vi "ShowLifetimeAndF2Image.vi"(2 "Path":refnum<vi>, 5 "threshold (min)":u16, 6 "notes 2":refnum<vi>) -> ()   [LabVIEW 2009]
panel:
  in  "save tau":bool
  in  "channel":u16(ring) items=["sum", "1", "2", "3", "4", "5", "6", "7", "8"]
  in  "draw F2 image":bool caption="display F2 image"
  in  "display tau image":bool
  in  "Color Palette F2-image":T1(ring)
  in  "min. F2 Value":sgl min=0 max=1 format="%.2f"
  in  "max. F2 Value":sgl=1.0 min=0 max=1 format="%.2f"
  in  "min. tau Value":dbl min=0.0 format="%.2f"
  in  "max. tau Value":dbl=10.0 min=0.0 format="%.2f"
  in  "Color Palette lifetime":T1(ring)
  in  "notes":string
  out "Ampel":cluster{"RED":bool, "YELLOW":bool, "GREEN":bool}
  in  "F2-channel":u8=2 min=1 max=16 step=1
  in  "Export":bool
  in  "stop":bool
  in  "plane":i32
  # "t"
  # "Fx"
  # "channel"
  # "S channel"
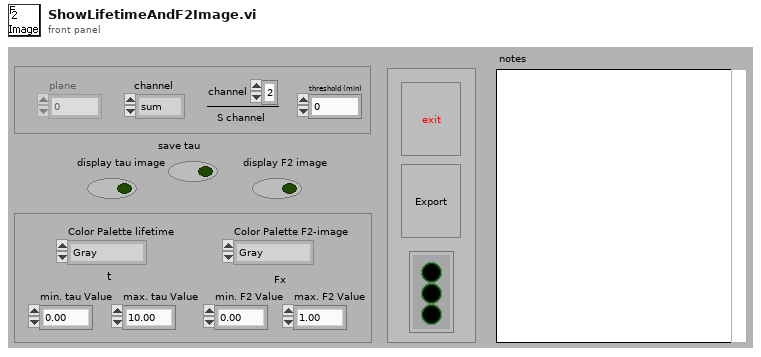
[diagram p1: front panel]
types:
  T1 = enum32{"Gray", "Binary", "Gradient", "Rainbow", "Temperature"}
  T2 = enum16{"create", "Input", "draw", "colorpal", "dump", "Get"}
  T3 = enum16{"create", "Input", "draw", "colorpal", "dump"}
  T4 = enum16{"ini", "get", "change", "export", "draw", "dump", "kill", "colorpal"}
  T5 = enum16{"create", "Input", "draw", "colorpal", "dump", "Get", "kill"}
  T6 = enum16{"create", "Input", "draw", "colorpal", "dump", "get", "kill"}
  T7 = enum16{"create", "Input", "draw", "colorpal", "dump", "get"}
  T8 = typedef "Settings.ctl" = cluster{"threshold":cluster{"max":u32, "min":u32}, "RGB or false color":bool, "16bit":bool, "log/lin axis":u16, "spotsize button":bool, "Pixelsize":u16, "autoscale x":bool, "autoscale y":bool, "correlation":bool, "ADC-Resolution":i32, "F2-lifetime":cluster{"display tau":bool, "display F2":bool, "Palette Number lifetime":enum32{"Gray", "Binary", "Gradient", "Rainbow", "Temperature"}, "Palette Number F2":enum32{"Gray", "Binary", "Gradient", "Rainbow", "Temperature"}, "max tau-Value":dbl, "min tau-Value":dbl, "max F2-Value":dbl, "min F2-Value":dbl}, "TAC-Window 1":u16, "TAC-Window 2":u16, "false color palette":cluster{"1":u32, "2":u32, "3":u32, "4":u32, "5":u32, "6":u32, "7":u32, "8":u32, "8 2":u32, "8 3":u32, "8 4":u32, "8 5":u32}}
  T9 = typedef "FIFOSettings_BH.ctt" = cluster{"Measurement":cluster{"Binning (ms)":sgl, "External Trigger Condition":u16, "Stop Condition:":u16, "Stop Count":dbl, "Buffer Size (Photons)":u16, "No of Channels":u16, "Ext Latch Delay":i16}, "ADC":cluster{"Module":u16, "ADC Resolution":i32, "Dither Range":i16, "Count Increment":i16, "Macro Time Clock":i16}, "SYNC":cluster{"SYNC ZC Level (mV)":sgl, "SYNC Freq Divider":i16, "SYNC Holdoff (ns)":sgl, "SYNC Threshold (mV)":sgl}, "TAC":cluster{"TAC Range (ns)":sgl, "TAC Gain":i16, "TAC Offset (%)":sgl, "TAC Limit Low (%)":sgl, "TAC Limit High (%)":sgl}, "CFD":cluster{"CFD Limit Low (mV)":sgl, "CFD Limit High (mV)":sgl, "CFD ZC Level (mV)":sgl, "CFD Holdoff (ns)":sgl}}
  T10 = typedef "ImageSettings.ctt" = cluster{"Start Position (µm)":cluster{"x":dbl, "y":dbl, "z":dbl}, "End Position (µm)":cluster{"x":dbl, "y":dbl, "z":dbl}, "Image Resolution (nm/pixel)":cluster{"x":dbl, "y":dbl, "z":dbl}, "Image Size (µm)":cluster{"x":dbl, "y":dbl, "z":dbl}, "Image Size (pixel)":cluster{"x":u32, "y":u32, "z":u32}, "Time Resolution\n(ms/pixel)":dbl, "1st Axis":u16, "2nd Axis":u16, "Retrace":bool, "Estimated Time":string}
  T11 = typedef "IMAQ Image.ctl" = refnum<image>
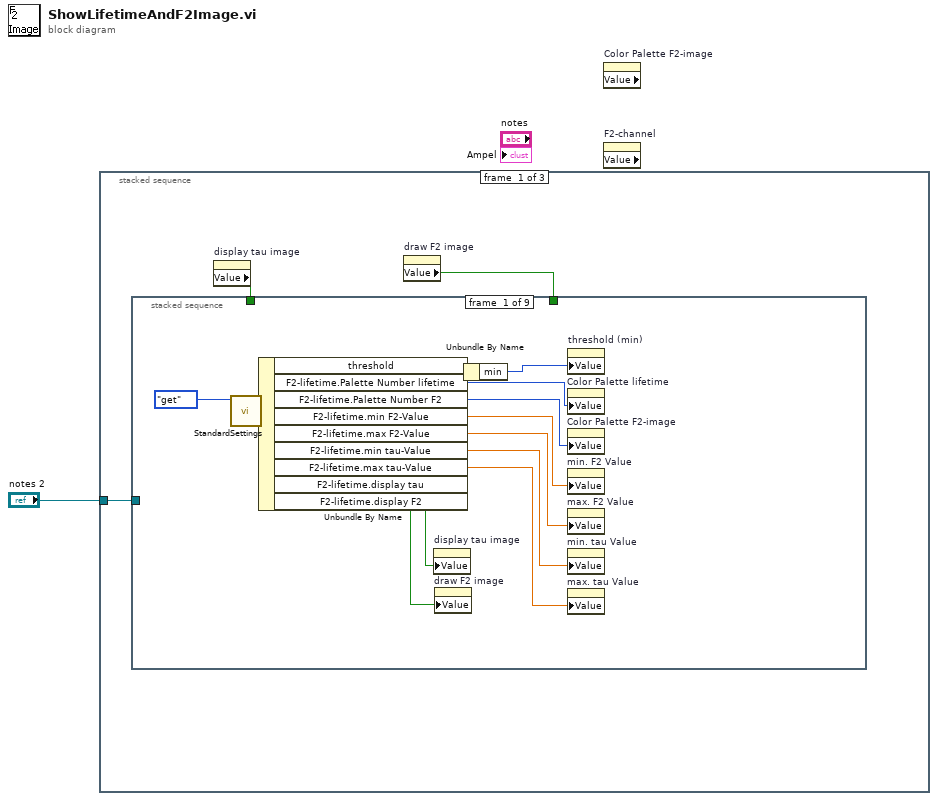
[diagram p0: block diagram]
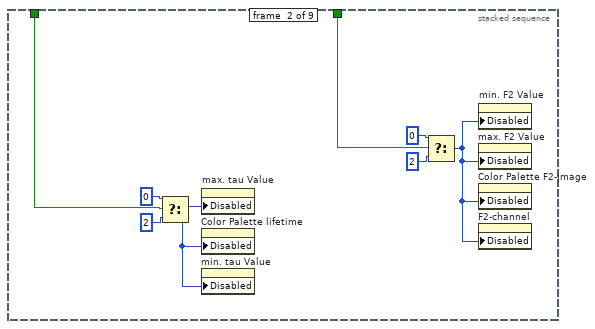
[diagram p2: hidden frame]
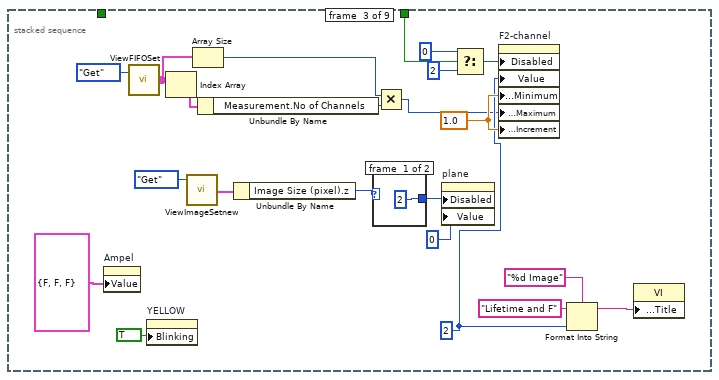
[diagram p3: hidden frame]
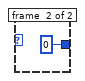
[diagram p4: hidden frame]
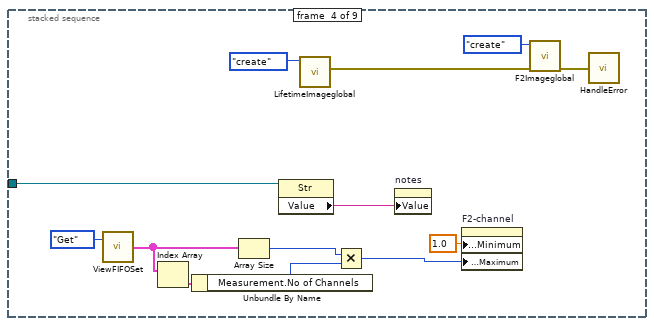
[diagram p5: hidden frame]
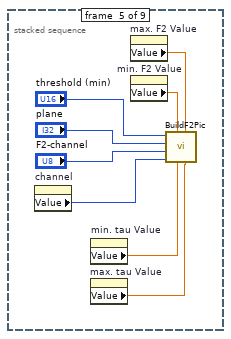
[diagram p6: hidden frame]
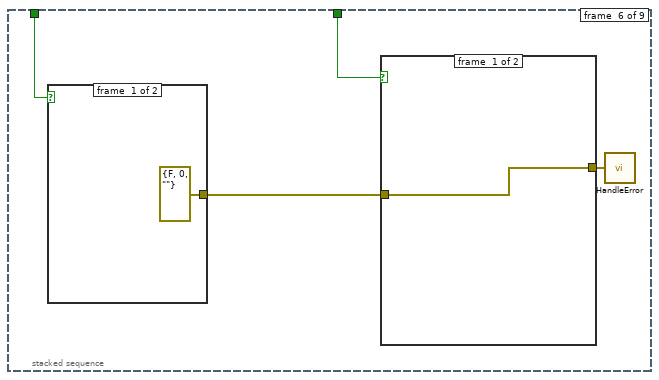
[diagram p7: hidden frame]
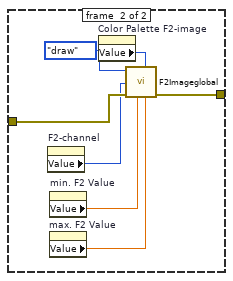
[diagram p8: hidden frame]
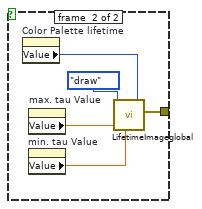
[diagram p9: hidden frame]
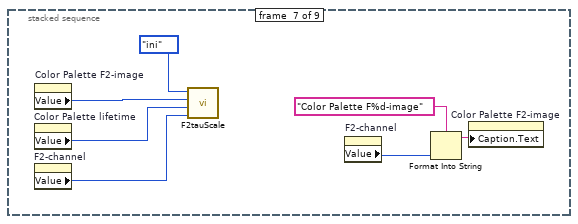
[diagram p10: hidden frame]
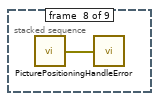
[diagram p11: hidden frame]
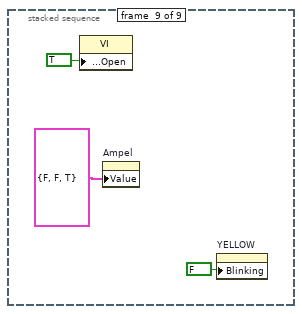
[diagram p12: hidden frame]
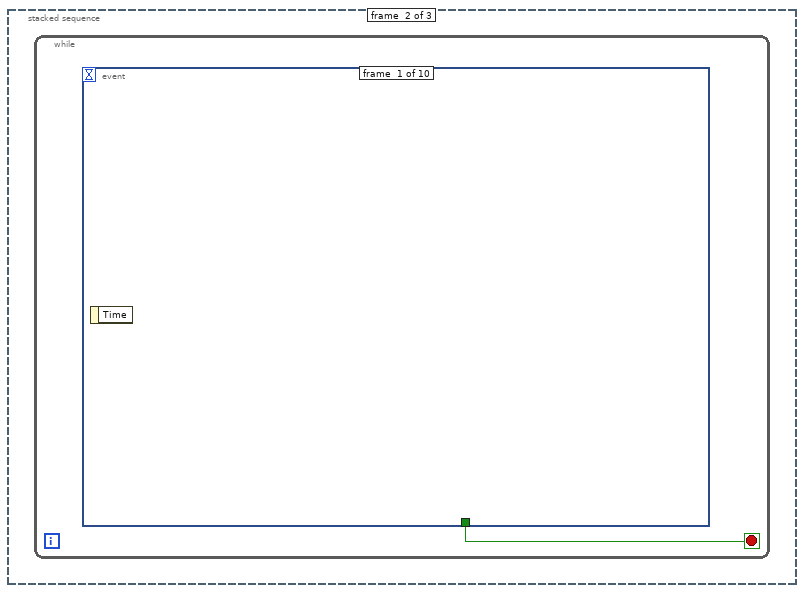
[diagram p13: hidden frame]
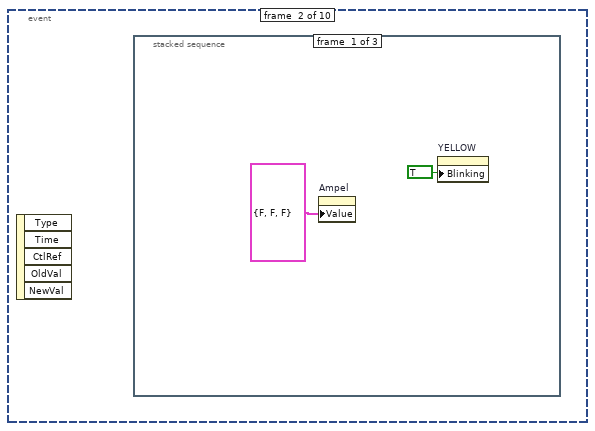
[diagram p14: hidden frame]
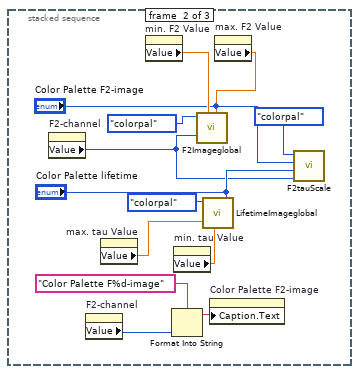
[diagram p15: hidden frame]
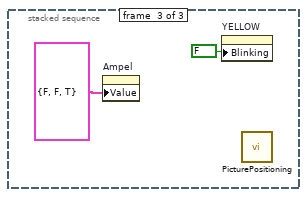
[diagram p16: hidden frame]
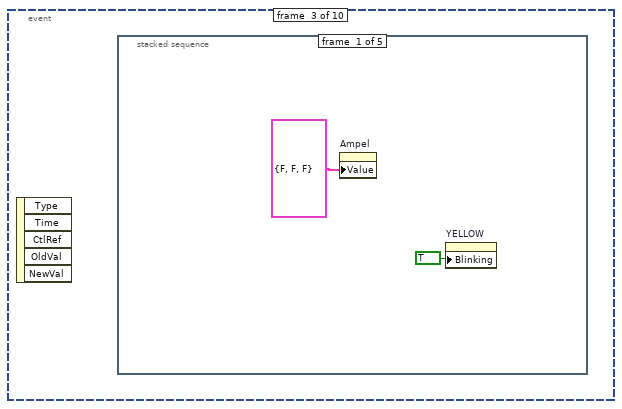
[diagram p17: hidden frame]
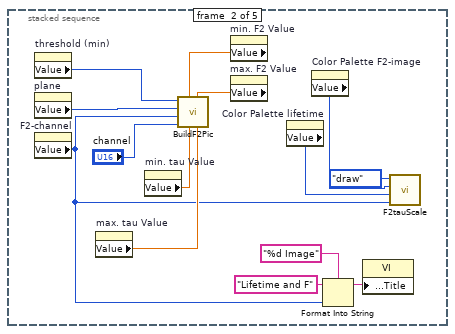
[diagram p18: hidden frame]
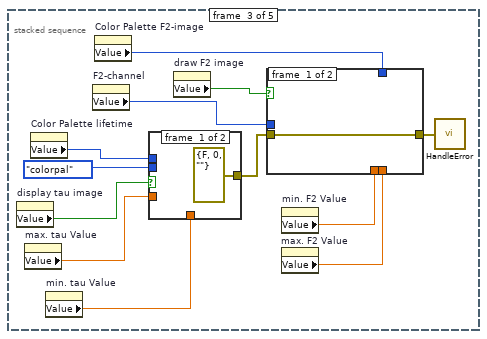
[diagram p19: hidden frame]
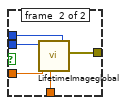
[diagram p20: hidden frame]
diagram:
  n1 = stacked-sequence {
    tunnel: "notes 2" -> [w4 _ w350]
    frame #0 {
      n2 = property on="display tau image" class="Bool (strict)"() -> ("Value"=w3:bool)  [unwired: 2 in, 2 out]
      n3 = property on="draw F2 image" class="Bool (strict)"() -> ("Value"=w2:bool)  [unwired: 2 in, 2 out]
      n4 = stacked-sequence {
        tunnel: w4 -> [_ _ _ w56 _ _ _ _ _]
        tunnel: w3 -> [_ w18 _ _ _ w72 _ _ _]
        tunnel: w2 -> [_ w17 w31 _ _ w70 _ _ _]
        frame #0 {
          n5 = call "StandardSettings.vi"("Enum"=enum16{"Load", "get", "Save", "set"}."get") -> ("StandardSettings"=w15:T8)  [unwired: 4 in]
          n6 = Unbundle By Name(w15) -> ("threshold"=w6:cluster{"max":u32, "min":u32}, "F2-lifetime.Palette Number lifetime"=w14:T1, "F2-lifetime.Palette Number F2"=w13:T1, "F2-lifetime.min F2-Value"=w12:dbl, "F2-lifetime.max F2-Value"=w11:dbl, "F2-lifetime.min tau-Value"=w10:dbl, "F2-lifetime.max tau-Value"=w9:dbl, "F2-lifetime.display tau"=w8:bool, "F2-lifetime.display F2"=w7:bool)
          n7 = property on="display tau image" class="Bool (strict)"("Value"=w8) -> ()  [unwired: 2 in, 2 out]
          n8 = property on="draw F2 image" class="Bool (strict)"("Value"=w7) -> ()  [unwired: 2 in, 2 out]
          n9 = Unbundle By Name(w6) -> ("min"=w5:u32)
          n10 = property on="threshold (min)" class="DigNum (strict)"("Value"=w5) -> ()  [unwired: 2 in, 2 out]
          n11 = property on="Color Palette lifetime" class="Enum (strict)"("Value"=w14) -> ()  [unwired: 2 in, 2 out]
          n12 = property on="Color Palette F2-image" class="Enum (strict)"("Value"=w13) -> ()  [unwired: 2 in, 2 out]
          n13 = property on="min. F2 Value" class="DigNum (strict)"("Value"=w12) -> ()  [unwired: 2 in, 2 out]
          n14 = property on="max. F2 Value" class="DigNum (strict)"("Value"=w11) -> ()  [unwired: 2 in, 2 out]
          n15 = property on="min. tau Value" class="DigNum (strict)"("Value"=w10) -> ()  [unwired: 2 in, 2 out]
          n16 = property on="max. tau Value" class="DigNum (strict)"("Value"=w9) -> ()  [unwired: 2 in, 2 out]
        }
        frame #1 {
          n17 = Select(t=0, s=w18, f=2) -> (s? t:f=w19:i32)
          n18 = property on="max. tau Value" class="DigNum (strict)"("Disabled"=w19) -> ()  [unwired: 2 in, 2 out]
          n19 = property on="Color Palette lifetime" class="Enum (strict)"("Disabled"=w19) -> ()  [unwired: 2 in, 2 out]
          n20 = property on="min. tau Value" class="DigNum (strict)"("Disabled"=w19) -> ()  [unwired: 2 in, 2 out]
          n21 = Select(t=0, s=w17, f=2) -> (s? t:f=w22:i32)
          n22 = property on="min. F2 Value" class="DigNum (strict)"("Disabled"=w22) -> ()  [unwired: 2 in, 2 out]
          n23 = property on="max. F2 Value" class="DigNum (strict)"("Disabled"=w22) -> ()  [unwired: 2 in, 2 out]
          n24 = property on="Color Palette F2-image" class="Enum (strict)"("Disabled"=w22) -> ()  [unwired: 2 in, 2 out]
          n25 = property on="F2-channel" class="DigNum (strict)"("Disabled"=w22) -> ()  [unwired: 2 in, 2 out]
        }
        frame #2 {
          w41 = 1.0 ("Data Range:Minimum")
          w38 = u8 2 ("F2-channel")
          n26 = property on="Ampel" class="Cluster (strict)"("Value"=cluster{"RED":bool, "YELLOW":bool, "GREEN":bool} {"RED"=FALSE, "YELLOW"=FALSE, "GREEN"=FALSE} ("Ampel")) -> ()  [unwired: 2 in, 2 out]
          n27 = call "ViewFIFOSet.vi"("Enum"=enum16{"Display", "change", "Get", "Set"}."Get") -> ("FIFO Settings (Array)"=w28:T9[])  [unwired: 1 in]
          n28 = property on="YELLOW" class="Boolean (strict)"("Blinking"=TRUE) -> ()  [unwired: 2 in, 2 out]
          n29 = Index Array(array=w28) -> (element=w29:T9)  [unwired: 1 in]
          n30 = call "ViewImageSetnew.vi"("action"=enum16{"Display", "change", "Get", "Set"}."Get" ("Enum")) -> ("Image Settings"=w44:T10)  [unwired: 2 in]
          n31 = Array Size(array=w28) -> (size(s)=w26:i32)
          n32 = Unbundle By Name(w29) -> ("Measurement.No of Channels"=w27:u16)
          n33 = Unbundle By Name(w44) -> ("Image Size (pixel).z"=w43:u32)
          n34 = case shown="1, Default" w43 {
            tunnel: [u8 2 u8 0] -> w42
            frame #0 {
            }
            frame #1 {
            }
          }
          n35 = Multiply(x=w26, y=w27) -> (x*y=w25:i32)
          n36 = property on="plane" class="DigNum (strict)"("Disabled"=w42, "Value"=0 ("plane")) -> ()  [unwired: 2 in, 2 out]
          n37 = Select(t=u8 0, s=w31, f=u8 2) -> (s? t:f=w35:u8)
          n38 = property on="F2-channel" class="DigNum (strict)"("Disabled"=w35, "Value"=w38, "Data Entry Limits:Minimum"=w41, "Data Entry Limits:Maximum"=w25, "Data Entry Limits:Increment"=w41) -> ()  [unwired: 2 in, 2 out]
          n39 = Format Into String(format string="%d Image", initial string="Lifetime and F", w38) -> (resulting string=w36:string)  [unwired: 1 in, 1 out]
          n40 = property class="VI"("Front Panel Window:Title"=w36) -> ()  [unwired: 2 in, 2 out]
        }
        frame #3 {
          n41 = call "ViewFIFOSet.vi"("Enum"=enum16{"Display", "change", "Get", "Set"}."Get") -> ("FIFO Settings (Array)"=w53:T9[])  [unwired: 1 in]
          n42 = Index Array(array=w53) -> (element=w52:T9)  [unwired: 1 in]
          n43 = Unbundle By Name(w52) -> ("Measurement.No of Channels"=w51:u16)
          n44 = Array Size(array=w53) -> (size(s)=w50:i32)
          n45 = property class="Str"(reference=w56) -> ("Value"=w57:string)  [unwired: 1 in, 2 out]
          n46 = call "LifetimeImageglobal.vi"("Enum"=T3."create") -> ("error out"=w61:errorcluster)  [unwired: 5 in, 2 out]
          n47 = Multiply(x=w50, y=w51) -> (x*y=w49:i32)
          n48 = property on="notes" class="String"("Value"=w57) -> ()  [unwired: 2 in, 2 out]
          n49 = property on="F2-channel" class="Digital (strict)"("Data Entry Limits:Minimum"=1.0 ("Data Range:Minimum"), "Data Entry Limits:Maximum"=w49) -> ()  [unwired: 2 in, 2 out]
          n50 = call "F2Imageglobal.vi"("error in"=w61, "Enum"=T2."create") -> ("error out"=w60:errorcluster)  [unwired: 7 in, 2 out]
          n51 = call "HandleError.vi"("error in (no error)"=w60) -> ()
        }
        frame #4 {
          n52 = property on="channel" class="Ring (strict)"() -> ("Value"=w62:u16)  [unwired: 2 in, 2 out]
          n53 = property on="min. tau Value" class="Digital (strict)"() -> ("Value"=w63:dbl)  [unwired: 2 in, 2 out]
          n54 = property on="max. tau Value" class="DigNum (strict)"() -> ("Value"=w64:dbl)  [unwired: 2 in, 2 out]
          n55 = property on="max. F2 Value" class="DigNum (strict)"() -> ("Value"=w66:sgl)  [unwired: 2 in, 2 out]
          n56 = property on="min. F2 Value" class="DigNum (strict)"() -> ("Value"=w65:sgl)  [unwired: 2 in, 2 out]
          n57 = call "BuildF2Pic.vi"("max tau"=w64, "max F2"=w66, "min tau"=w63, "min F2"=w65, "channel"=w62, "F2-channel"="F2-channel", "plane"="plane", "threshold"="threshold (min)") -> ()  [unwired: 4 in]
        }
        frame #5 {
          n58 = case shown="True" w72 {
            tunnel: [errorcluster {"status"=FALSE, "code"=0, "source"=""} ("error out") w87] -> w73
            frame #0 {
            }
            frame #1 {
              n59 = property on="Color Palette lifetime" class="Enum (strict)"() -> ("Value"=w85:T1)  [unwired: 2 in, 2 out]
              n60 = property on="max. tau Value" class="DigNum (strict)"() -> ("Value"=w84:dbl)  [unwired: 2 in, 2 out]
              n61 = property on="min. tau Value" class="Digital (strict)"() -> ("Value"=w83:dbl)  [unwired: 2 in, 2 out]
              n62 = call "LifetimeImageglobal.vi"("Palette Number (gray)"=w85, "min tau value"=w83, "max tau value"=w84, "Enum"=T3."draw") -> ("error out"=w87:errorcluster)  [unwired: 2 in, 2 out]
            }
          }
          n63 = case shown="True" w70 {
            tunnel: w73 -> [w74 w81]
            tunnel: [w74 w75] -> w71
            frame #0 {
            }
            frame #1 {
              n64 = property on="F2-channel" class="DigNum (strict)"() -> ("Value"=w79:u8)  [unwired: 2 in, 2 out]
              n65 = property on="min. F2 Value" class="DigNum (strict)"() -> ("Value"=w77:sgl)  [unwired: 2 in, 2 out]
              n66 = property on="max. F2 Value" class="DigNum (strict)"() -> ("Value"=w76:sgl)  [unwired: 2 in, 2 out]
              n67 = property on="Color Palette F2-image" class="Enum (strict)"() -> ("Value"=w78:T1)  [unwired: 2 in, 2 out]
              n68 = call "F2Imageglobal.vi"("max"=w76, "Palette Number (gray)"=w78, "min"=w77, "error in"=w81, "Fx channel"=w79, "Enum"=T2."draw") -> ("error out"=w75:errorcluster)  [unwired: 3 in, 2 out]
            }
          }
          n69 = call "HandleError.vi"("error in (no error)"=w71) -> ()
        }
        frame #6 {
          n70 = property on="Color Palette F2-image" class="Enum (strict)"() -> ("Value"=w91:T1)  [unwired: 2 in, 2 out]
          n71 = property on="Color Palette lifetime" class="Enum (strict)"() -> ("Value"=w90:T1)  [unwired: 2 in, 2 out]
          n72 = property on="F2-channel" class="Digital (strict)"() -> ("Value"=w89:u8)  [unwired: 2 in, 2 out]
          n73 = call "F2tauScale.vi"("F2 channel"=w89, "Palette tau"=w90, "Palette F2"=w91, "Enum"=T4."ini") -> ()  [unwired: 3 in, 5 out]
          n74 = property on="F2-channel" class="DigNum (strict)"() -> ("Value"=w92:u8)  [unwired: 2 in, 2 out]
          n75 = Format Into String(format string="Color Palette F%d-image", w92) -> (resulting string=w94:string)  [unwired: 2 in, 1 out]
          n76 = property on="Color Palette F2-image" class="Enum (strict)"("Caption.Text"=w94) -> ()  [unwired: 2 in, 2 out]
        }
        frame #7 {
          n77 = call "PicturePositioning.vi"() -> ("error out"=w95:errorcluster)
          n78 = call "HandleError.vi"("error in (no error)"=w95) -> ()
        }
        frame #8 {
          n79 = property class="VI"("Front Panel Window:Open"=TRUE) -> ()  [unwired: 2 in, 2 out]
          n80 = property on="Ampel" class="Cluster (strict)"("Value"=cluster{"RED":bool, "YELLOW":bool, "GREEN":bool} {"RED"=FALSE, "YELLOW"=FALSE, "GREEN"=TRUE} ("Ampel")) -> ()  [unwired: 2 in, 2 out]
          n81 = property on="YELLOW" class="Boolean (strict)"("Blinking"=FALSE) -> ()  [unwired: 2 in, 2 out]
        }
      }
    }
    frame #1 {
      n82 = while {
        stop <- w99 stop-if-true
        n83 = event shown="[6] \"save tau\": Value Change" {
          selector: _ -> [_ _ _ _ _ _ _ _ _ _]
          dyn-events: _ -> [_ _ _ _ _ _ _ _ _ _]
          timeout: _ -> [_ _ _ _ _ _ _ _ _ _]
          tunnel: [_ _ _ _ _ _ _ _ w334 TRUE] -> w99
          event #0 {
            n84 = event-data() -> ()  [unwired: 1 in, 1 out]
          }
          event #1 {
            n85 = event-data() -> ()  [unwired: 1 in, 5 out]
            n86 = stacked-sequence {
              frame #0 {
                n87 = property on="Ampel" class="Cluster (strict)"("Value"=cluster{"RED":bool, "YELLOW":bool, "GREEN":bool} {"RED"=FALSE, "YELLOW"=FALSE, "GREEN"=FALSE} ("Ampel")) -> ()  [unwired: 2 in, 2 out]
                n88 = property on="YELLOW" class="Boolean (strict)"("Blinking"=TRUE) -> ()  [unwired: 2 in, 2 out]
              }
              frame #1 {
                n89 = property on="F2-channel" class="DigNum (strict)"() -> ("Value"=w103:u8)  [unwired: 2 in, 2 out]
                n90 = property on="F2-channel" class="DigNum (strict)"() -> ("Value"=w106:u8)  [unwired: 2 in, 2 out]
                n91 = property on="max. tau Value" class="DigNum (strict)"() -> ("Value"=w112:dbl)  [unwired: 2 in, 2 out]
                n92 = property on="min. F2 Value" class="DigNum (strict)"() -> ("Value"=w110:sgl)  [unwired: 2 in, 2 out]
                n93 = Format Into String(format string="Color Palette F%d-image", w106) -> (resulting string=w108:string)  [unwired: 2 in, 1 out]
                n94 = property on="min. tau Value" class="Digital (strict)"() -> ("Value"=w111:dbl)  [unwired: 2 in, 2 out]
                n95 = call "LifetimeImageglobal.vi"("Palette Number (gray)"="Color Palette lifetime", "min tau value"=w111, "max tau value"=w112, "Enum"=T3."colorpal") -> ()  [unwired: 2 in, 3 out]
                n96 = property on="Color Palette F2-image" class="Enum (strict)"("Caption.Text"=w108) -> ()  [unwired: 2 in, 2 out]
                n97 = property on="max. F2 Value" class="DigNum (strict)"() -> ("Value"=w109:sgl)  [unwired: 2 in, 2 out]
                n98 = call "F2Imageglobal.vi"("max"=w109, "Palette Number (gray)"="Color Palette F2-image", "min"=w110, "Fx channel"=w103, "Enum"=T2."colorpal") -> ()  [unwired: 4 in, 3 out]
                n99 = call "F2tauScale.vi"("F2 channel"=w103, "Palette tau"="Color Palette lifetime", "Palette F2"="Color Palette F2-image", "Enum"=T4."colorpal") -> ()  [unwired: 3 in, 5 out]
              }
              frame #2 {
                n100 = property on="Ampel" class="Cluster (strict)"("Value"=cluster{"RED":bool, "YELLOW":bool, "GREEN":bool} {"RED"=FALSE, "YELLOW"=FALSE, "GREEN"=TRUE} ("Ampel")) -> ()  [unwired: 2 in, 2 out]
                n101 = property on="YELLOW" class="Boolean (strict)"("Blinking"=FALSE) -> ()  [unwired: 2 in, 2 out]
                n102 = call "PicturePositioning.vi"() -> ()  [unwired: 1 out]
              }
            }
          }
          event #2 {
            n103 = event-data() -> ()  [unwired: 1 in, 5 out]
            n104 = stacked-sequence {
              frame #0 {
                n105 = property on="Ampel" class="Cluster (strict)"("Value"=cluster{"RED":bool, "YELLOW":bool, "GREEN":bool} {"RED"=FALSE, "YELLOW"=FALSE, "GREEN"=FALSE} ("Ampel")) -> ()  [unwired: 2 in, 2 out]
                n106 = property on="YELLOW" class="Boolean (strict)"("Blinking"=TRUE) -> ()  [unwired: 2 in, 2 out]
              }
              frame #1 {
                n107 = property on="threshold (min)" class="DigNum (strict)"() -> ("Value"=w132:u16)  [unwired: 2 in, 2 out]
                n108 = property on="plane" class="DigNum (strict)"() -> ("Value"=w131:i32)  [unwired: 2 in, 2 out]
                n109 = property on="F2-channel" class="DigNum (strict)"() -> ("Value"=w120:u8)  [unwired: 2 in, 2 out]
                n110 = property on="max. tau Value" class="DigNum (strict)"() -> ("Value"=w130:dbl)  [unwired: 2 in, 2 out]
                n111 = property on="min. tau Value" class="Digital (strict)"() -> ("Value"=w129:dbl)  [unwired: 2 in, 2 out]
                n112 = property on="min. F2 Value" class="DigNum (strict)"() -> ("Value"=w127:sgl)  [unwired: 2 in, 2 out]
                n113 = property on="max. F2 Value" class="DigNum (strict)"() -> ("Value"=w128:sgl)  [unwired: 2 in, 2 out]
                n114 = call "BuildF2Pic.vi"("max tau"=w130, "max F2"=w128, "min tau"=w129, "min F2"=w127, "channel"="channel", "F2-channel"=w120, "plane"=w131, "threshold"=w132) -> ()  [unwired: 4 in]
                n115 = property on="Color Palette lifetime" class="Enum (strict)"() -> ("Value"=w123:T1)  [unwired: 2 in, 2 out]
                n116 = property on="Color Palette F2-image" class="Enum (strict)"() -> ("Value"=w121:T1)  [unwired: 2 in, 2 out]
                n117 = Format Into String(format string="%d Image", initial string="Lifetime and F", w120) -> (resulting string=w124:string)  [unwired: 1 in, 1 out]
                n118 = property class="VI"("Front Panel Window:Title"=w124) -> ()  [unwired: 2 in, 2 out]
                n119 = call "F2tauScale.vi"("F2 channel"=w120, "Palette tau"=w123, "Palette F2"=w121, "Enum"=T4."draw") -> ()  [unwired: 3 in, 5 out]
              }
              frame #2 {
                n120 = property on="display tau image" class="Bool (strict)"() -> ("Value"=w133:bool)  [unwired: 2 in, 2 out]
                n121 = property on="max. tau Value" class="DigNum (strict)"() -> ("Value"=w138:dbl)  [unwired: 2 in, 2 out]
                n122 = property on="Color Palette lifetime" class="Enum (strict)"() -> ("Value"=w143:T1)  [unwired: 2 in, 2 out]
                n123 = property on="min. tau Value" class="Digital (strict)"() -> ("Value"=w139:dbl)  [unwired: 2 in, 2 out]
                n124 = property on="F2-channel" class="DigNum (strict)"() -> ("Value"=w140:u8)  [unwired: 2 in, 2 out]
                n125 = property on="Color Palette F2-image" class="Enum (strict)"() -> ("Value"=w142:T1)  [unwired: 2 in, 2 out]
                n126 = case shown="False" w133 {
                  tunnel: [errorcluster {"status"=FALSE, "code"=0, "source"=""} ("error out") w150] -> w144
                  tunnel: w143 -> [_ w149]
                  tunnel: T3."colorpal" ("Enum") -> [_ w148]
                  tunnel: w139 -> [_ w147]
                  tunnel: w138 -> [_ w146]
                  frame #0 {
                  }
                  frame #1 {
                    n127 = call "LifetimeImageglobal.vi"("Palette Number (gray)"=w149, "min tau value"=w147, "max tau value"=w146, "Enum"=w148) -> ("error out"=w150:errorcluster)  [unwired: 2 in, 2 out]
                  }
                }
                n128 = property on="draw F2 image" class="Bool (strict)"() -> ("Value"=w134:bool)  [unwired: 2 in, 2 out]
                n129 = property on="min. F2 Value" class="DigNum (strict)"() -> ("Value"=w137:sgl)  [unwired: 2 in, 2 out]
                n130 = property on="max. F2 Value" class="DigNum (strict)"() -> ("Value"=w136:sgl)  [unwired: 2 in, 2 out]
                n131 = case shown="True" w134 {
                  tunnel: w144 -> [w151 w158]
                  tunnel: w142 -> [_ w157]
                  tunnel: w140 -> [_ w155]
                  tunnel: w137 -> [_ w154]
                  tunnel: w136 -> [_ w153]
                  tunnel: [w151 w152] -> w135
                  frame #0 {
                  }
                  frame #1 {
                    n132 = call "F2Imageglobal.vi"("max"=w153, "Palette Number (gray)"=w157, "min"=w154, "error in"=w158, "Fx channel"=w155, "Enum"=T2."colorpal") -> ("error out"=w152:errorcluster)  [unwired: 3 in, 2 out]
                  }
                }
                n133 = call "HandleError.vi"("error in (no error)"=w135) -> ()
              }
              frame #3 {
                n134 = property on="F2-channel" class="DigNum (strict)"() -> ("Value"=w168:u8)  [unwired: 2 in, 2 out]
                n135 = property on="F2-channel" class="DigNum (strict)"() -> ("Value"=w159:u8)  [unwired: 2 in, 2 out]
                n136 = Format Into String(format string=". F%d Value", w168) -> (resulting string=w166:string)  [unwired: 2 in, 1 out]
                n137 = Format Into String(format string="Color Palette F%d-image", w159) -> (resulting string=w161:string)  [unwired: 2 in, 1 out]
                n138 = property on="Color Palette F2-image" class="Enum (strict)"("Caption.Text"=w161) -> ()  [unwired: 2 in, 2 out]
                n139 = Concatenate Strings("min" ("string"), w166) -> (w163:string)
                n140 = Concatenate Strings("max" ("string"), w166) -> (w162:string)
                n141 = property on="min. F2 Value" class="DigNum (strict)"("Caption.Text"=w163) -> ()  [unwired: 2 in, 2 out]
                n142 = property on="max. F2 Value" class="DigNum (strict)"("Caption.Text"=w162) -> ()  [unwired: 2 in, 2 out]
              }
              frame #4 {
                n143 = property on="Ampel" class="Cluster (strict)"("Value"=cluster{"RED":bool, "YELLOW":bool, "GREEN":bool} {"RED"=FALSE, "YELLOW"=FALSE, "GREEN"=TRUE} ("Ampel")) -> ()  [unwired: 2 in, 2 out]
                n144 = call "PicturePositioning.vi"() -> ()  [unwired: 1 out]
                n145 = property on="YELLOW" class="Boolean (strict)"("Blinking"=FALSE) -> ()  [unwired: 2 in, 2 out]
              }
            }
          }
          event #3 {
            n146 = event-data() -> ("CtlRef"=w172:refnum<vi>, "NewVal"=w171:bool)  [unwired: 1 in, 3 out]
            n147 = stacked-sequence {
              seq-local: [_ w175 _ _] -> [_ _ w213 _]
              seq-local: [_ w174 _ _] -> [_ _ w212 _]
              seq-local: [_ w173 _ _] -> [_ _ w211 _]
              tunnel: w172 -> [_ w186 _ _]
              tunnel: w171 -> [_ w180 _ _]
              frame #0 {
              }
              frame #1 {
                n148 = control-ref of="display tau image"() -> (w185:refnum<vi>)
                n149 = call "StandardSettings.vi"("Enum"=enum16{"Load", "get", "Save", "set"}."get") -> ("StandardSettings"=w177:T8)  [unwired: 4 in]
                n150 = Select(t=0, s=w180, f=2) -> (s? t:f=w181:i32)
                n151 = Equal?(x=w185, y=w186) -> (x = y?=w182:bool)
                n152 = case shown="False" w182 {
                  tunnel: w181 -> [w198 w210]
                  tunnel: w180 -> [w192 w204]
                  tunnel: w177 -> [w194 w206]
                  tunnel: [w193 w205] -> w176
                  tunnel: [w189 w201] -> w175
                  tunnel: [w188 w200] -> w174
                  tunnel: [w187 w199] -> w173
                  frame #0 {
                    n153 = Bundle By Name(cluster=w194, "F2-lifetime.display F2"=w192) -> (w193:T8)
                    n154 = Select(t=T5."draw" ("Enum"), s=w192, f=T5."kill" ("Enum")) -> (s? t:f=w195:T5)
                    n155 = property on="min. F2 Value" class="DigNum (strict)"("Disabled"=w198) -> ("Value"=w190:sgl)  [unwired: 2 in, 2 out]
                    n156 = property on="Color Palette F2-image" class="Enum (strict)"("Disabled"=w198) -> ("Value"=w189:T1)  [unwired: 2 in, 2 out]
                    n157 = property on="F2-channel" class="DigNum (strict)"("Disabled"=w198) -> ("Value"=w187:u8)  [unwired: 2 in, 2 out]
                    n158 = property on="max. F2 Value" class="DigNum (strict)"("Disabled"=w198) -> ("Value"=w191:sgl)  [unwired: 2 in, 2 out]
                    n159 = call "F2Imageglobal.vi"("max"=w191, "Palette Number (gray)"=w189, "min"=w190, "Fx channel"=w187, "Enum"=w195) -> ()  [unwired: 4 in, 3 out]
                    n160 = property on="Color Palette lifetime" class="Enum (strict)"() -> ("Value"=w188:T1)  [unwired: 2 in, 2 out]
                  }
                  frame #1 {
                    n161 = Bundle By Name(cluster=w206, "F2-lifetime.display tau"=w204) -> (w205:T8)
                    n162 = property on="min. tau Value" class="DigNum (strict)"("Disabled"=w210) -> ("Value"=w203:dbl)  [unwired: 2 in, 2 out]
                    n163 = property on="max. tau Value" class="DigNum (strict)"("Disabled"=w210) -> ("Value"=w202:dbl)  [unwired: 2 in, 2 out]
                    n164 = property on="Color Palette lifetime" class="Enum (strict)"("Disabled"=w210) -> ("Value"=w200:T1)  [unwired: 2 in, 2 out]
                    n165 = Select(t=T6."draw" ("Enum"), s=w204, f=T6."kill") -> (s? t:f=w207:T6)
                    n166 = call "LifetimeImageglobal.vi"("Palette Number (gray)"=w200, "min tau value"=w203, "max tau value"=w202, "Enum"=w207) -> ()  [unwired: 2 in, 3 out]
                    n167 = property on="Color Palette F2-image" class="Enum (strict)"() -> ("Value"=w201:T1)  [unwired: 2 in, 2 out]
                    n168 = property on="F2-channel" class="DigNum (strict)"() -> ("Value"=w199:u8)  [unwired: 2 in, 2 out]
                  }
                }
                n169 = call "StandardSettings.vi"("StandardSettings"=w176, "Enum"=enum16{"Load", "get", "Save", "set"}."set") -> ()  [unwired: 3 in, 1 out]
              }
              frame #2 {
                n170 = call "F2tauScale.vi"("F2 channel"=w211, "Palette tau"=w212, "Palette F2"=w213, "Enum"=T4."change") -> ()  [unwired: 3 in, 5 out]
              }
              frame #3 {
                n171 = call "PicturePositioning.vi"() -> ()  [unwired: 1 out]
              }
            }
          }
          event #4 {
            n172 = event-data() -> ()  [unwired: 1 in, 5 out]
            n173 = stacked-sequence {
              seq-local: [_ w221 _ _ _] -> [_ _ w233 _ _]
              seq-local: [_ _ w227 _ _] -> [_ _ _ _ _]
              seq-local: [_ _ w226 _ _] -> [_ _ _ _ _]
              frame #0 {
                n174 = property on="Ampel" class="Cluster (strict)"("Value"=cluster{"RED":bool, "YELLOW":bool, "GREEN":bool} {"RED"=FALSE, "YELLOW"=FALSE, "GREEN"=FALSE} ("Ampel")) -> ()  [unwired: 2 in, 2 out]
                n175 = property on="YELLOW" class="Boolean (strict)"("Blinking"=TRUE) -> ()  [unwired: 2 in, 2 out]
              }
              frame #1 {
                n176 = property on="F2-channel" class="DigNum (strict)"() -> ("Value"=w217:u8)  [unwired: 2 in, 2 out]
                n177 = Format Into String(initial string="F", w217) -> (resulting string=w219:string)  [unwired: 2 in, 1 out]
                n178 = Two Button Dialog(message="Which image?", 1:w219, 2:"lifetime" ("F button name (\"Cancel\")")) -> (T button?=w222:bool)
                n179 = Not(x=w222) -> (.not. x?=w221:bool)
              }
              frame #2 {
                n180 = property on="F2-channel" class="DigNum (strict)"() -> ("Value"=w228:u8)  [unwired: 2 in, 2 out]
                n181 = case shown="False" w233 {
                  tunnel: [w246 w253] -> w232
                  tunnel: [w239 w250] -> w226
                  tunnel: [w245 w252] -> w230
                  tunnel: [w242 w248] -> w229
                  tunnel: w228 -> [_ w249]
                  frame #0 {
                    n182 = property on="channel" class="Ring (strict)"() -> ("Value"=w238:u16)  [unwired: 2 in, 2 out]
                    n183 = Number To Decimal String(number=w238) -> (decimal integer string=w237:string)  [unwired: 1 in]
                    n184 = property on="Color Palette lifetime" class="Enum (strict)"() -> ("Value"=w245:T1)  [unwired: 2 in, 2 out]
                    n185 = Equal To 0?(x=w238) -> (x = 0?=w241:bool)
                    n186 = call "LifetimeImageglobal.vi"("Enum"=T7."get") -> ("title"=w240:string, "New Image"=w246:T11)  [unwired: 5 in, 1 out]
                    n187 = Select(t="sum", s=w241, f=w237) -> (s? t:f=w235:string)
                    n188 = call "F2tauScale.vi"("Enum"=T4."export") -> ("tauscale"=w242:T11)  [unwired: 6 in, 4 out]
                    n189 = Concatenate Strings(w240, " " ("string"), w235) -> (w239:string)
                  }
                  frame #1 {
                    n190 = property on="Color Palette F2-image" class="Enum (strict)"() -> ("Value"=w252:T1)  [unwired: 2 in, 2 out]
                    n191 = call "F2Imageglobal.vi"("Palette Number (gray)"=w252, "Enum"=T2."Get") -> ("String"=w250:string, "New Image"=w253:T11)  [unwired: 7 in, 1 out]
                    n192 = call "F2tauScale.vi"("F2 channel"=w249, "Enum"=T4."export") -> ("F2-scale"=w248:T11)  [unwired: 5 in, 4 out]
                  }
                }
                n193 = control-ref of="notes"() -> (w225:refnum<vi>)
                n194 = call "ExportPicture.vi"("Palette Number (gray)"=w230, "Image"=w232, "Image Scalebar"=w229, "name input"=w226, "Path"="Path", "notes 2"=w225) -> ("Numeric"=w227:i32, "error out"=w224:errorcluster)  [unwired: 1 in]
                n195 = call "HandleError.vi"("error in (no error)"=w224) -> ()
              }
              frame #3 {
                n196 = property on="Color Palette F2-image" class="Enum (strict)"() -> ("Value"=w257:T1)  [unwired: 2 in, 2 out]
                n197 = property on="Color Palette lifetime" class="Enum (strict)"() -> ("Value"=w256:T1)  [unwired: 2 in, 2 out]
                n198 = property on="F2-channel" class="DigNum (strict)"() -> ("Value"=w255:u8)  [unwired: 2 in, 2 out]
                n199 = call "F2tauScale.vi"("F2 channel"=w255, "Palette tau"=w256, "Palette F2"=w257, "Enum"=T4."change") -> ()  [unwired: 3 in, 5 out]
              }
              frame #4 {
                n200 = property on="Ampel" class="Cluster (strict)"("Value"=cluster{"RED":bool, "YELLOW":bool, "GREEN":bool} {"RED"=FALSE, "YELLOW"=FALSE, "GREEN"=TRUE} ("Ampel")) -> ()  [unwired: 2 in, 2 out]
                n201 = property on="YELLOW" class="Boolean (strict)"("Blinking"=FALSE) -> ()  [unwired: 2 in, 2 out]
                n202 = call "PicturePositioning.vi"() -> ()  [unwired: 1 out]
              }
            }
          }
          event #5 {
            n203 = event-data() -> ()  [unwired: 1 in, 5 out]
            n204 = property on="display tau image" class="Bool (strict)"() -> ("Value"=w260:bool)  [unwired: 2 in, 2 out]
            n205 = Max & Min(x="min. tau Value", y="max. tau Value") -> (max(x,y)=w261:dbl, min(x,y)=w262:dbl)
            n206 = Subtract(x=w261, y=w262) -> (x-y=w263:dbl)
            n207 = case shown="True" w260 {
              tunnel: w263 -> [_ w272]
              tunnel: w262 -> [_ w269]
              tunnel: w261 -> [_ w268]
              frame #0 {
              }
              frame #1 {
                n208 = call "tauImgValues.vi"("Set?"=FALSE) -> ("tau-values output"=w266:dbl[][])  [unwired: 1 in]
                n209 = Subtract(x=w266, y=w269) -> (x-y=w275:dbl[][])
                n210 = In Range and Coerce(upper limit=w272, x=w275, lower limit=0.0) -> (coerced(x)=w274:dbl[][])  [unwired: 1 out]
                n211 = Divide(x=255.0, y=w272) -> (x/y=w278:dbl)
                n212 = Multiply(x=w274, y=w278) -> (x*y=w280:dbl[][])
                n213 = To Unsigned Byte Integer(number=w280) -> (unsigned 8bit integer=w279:u8[][])
                n214 = property on="Color Palette lifetime" class="Enum (strict)"() -> ("Value"=w267:T1)  [unwired: 2 in, 2 out]
                n215 = call "LifetimeImageglobal.vi"("input Image array"=w279, "Enum"=T7."Input") -> ("error out"=w271:errorcluster)  [unwired: 4 in, 2 out]
                n216 = call "LifetimeImageglobal.vi"("Palette Number (gray)"=w267, "min tau value"=w269, "max tau value"=w268, "error in"=w271, "Enum"=T7."draw") -> ()  [unwired: 1 in, 3 out]
              }
            }
            n217 = property on="max. tau Value" class="DigNum (strict)"("Value"=w261) -> ()  [unwired: 2 in, 2 out]
            n218 = property on="min. tau Value" class="Digital (strict)"("Value"=w262) -> ()  [unwired: 2 in, 2 out]
          }
          event #6 {
            n219 = event-data() -> ()  [unwired: 1 in, 6 out]
            n220 = property on="max. tau Value" class="DigNum (strict)"() -> ("Value"=w305:dbl)  [unwired: 2 in, 2 out]
            n221 = property on="min. tau Value" class="Digital (strict)"() -> ("Value"=w306:dbl)  [unwired: 2 in, 2 out]
            n222 = call "sumofphotons.vi"("s"=FALSE) -> ("sum of photons out"=w297:u32[][][][])  [unwired: 1 in]
            n223 = call "tauImgValues.vi"("Set?"=FALSE) -> ("tau-values output"=w301:dbl[][])  [unwired: 1 in]
            n224 = Index Array(array=w297, index (dim 1)=0 ("disabled index (page)")) -> (element=w290:u32[][][])  [unwired: 3 in]
            n225 = Subtract(x=w301, y=w306) -> (x-y=w303:dbl[][])
            n226 = Array Size(array=w290) -> (size(s)=w296:i32[])
            n227 = Subtract(x=w305, y=w306) -> (x-y=w307:dbl)
            n228 = Index Array(array=w296, index #1=1 ("index (page)"), index #2=2 ("disabled index (row)")) -> (element #1=w292:i32, element #2=w293:i32)
            n229 = In Range and Coerce(upper limit=w307, x=w303, lower limit=0.0) -> (coerced(x)=w299:dbl[][])  [unwired: 1 out]
            n230 = Initialize Array(0.0 ("index (page)"), w292, w293) -> (w289:dbl[][])
            n231 = Array Size(array=w299) -> (size(s)=w300:i32[])
            n232 = Multiply Array Elements(1:w300) -> (0:w286:i32)
            n233 = for {
              tunnel: w290 -> [w310] mode=indexing
              shift-right: [w308] -> w287
              shift-left: w289 -> [w309]
              n234 = Add(x=w310, y=w309) -> (x+y=w308:dbl[][])
            }
            n235 = Reshape Array(w299, w286) -> (w284:dbl[])
            n236 = Reshape Array(w287, w286) -> (w285:dbl[])
            n237 = Build Array(w285, w284) -> (w283:dbl[][])
            n238 = call "Write To Spreadsheet File.vi"("transpose? (no:F)"=TRUE, "2D data"=w283) -> ()  [unwired: 6 in, 1 out]
          }
          event #7 {
            n239 = event-data() -> ()  [unwired: 1 in, 5 out]
            n240 = property on="draw F2 image" class="Bool (strict)"() -> ("Value"=w311:bool)  [unwired: 2 in, 2 out]
            n241 = Max & Min(x="max. F2 Value", y="min. F2 Value") -> (max(x,y)=w312:sgl, min(x,y)=w313:sgl)
            n242 = case shown="True" w311 {
              tunnel: w313 -> [_ w320]
              tunnel: w312 -> [_ w319]
              frame #0 {
              }
              frame #1 {
                n243 = call "F2ImgValues.vi"("Set?"=FALSE) -> ("F2-values"=w328:sgl[][])  [unwired: 1 in]
                n244 = Subtract(x=w328, y=w320) -> (x-y=w324:sgl[][])
                n245 = Subtract(x=w319, y=w320) -> (x-y=w325:sgl)
                n246 = In Range and Coerce(upper limit=w325, x=w324, lower limit=sgl 0.0 ("x")) -> (coerced(x)=w326:sgl[][])  [unwired: 1 out]
                n247 = Divide(x=sgl 255.0, y=w325) -> (x/y=w332:sgl)
                n248 = Multiply(x=w332, y=w326) -> (x*y=w331:sgl[][])
                n249 = property on="F2-channel" class="DigNum (strict)"() -> ("Value"=w318:u8)  [unwired: 2 in, 2 out]
                n250 = To Unsigned Byte Integer(number=w331) -> (unsigned 8bit integer=w330:u8[][])
                n251 = property on="Color Palette F2-image" class="Enum (strict)"() -> ("Value"=w317:T1)  [unwired: 2 in, 2 out]
                n252 = call "F2Imageglobal.vi"("input Image array"=w330, "Enum"=T2."Input") -> ("error out"=w322:errorcluster)  [unwired: 7 in, 2 out]
                n253 = call "F2Imageglobal.vi"("max"=w319, "Palette Number (gray)"=w317, "min"=w320, "error in"=w322, "Fx channel"=w318, "Enum"=T2."draw") -> ("error out"=w316:errorcluster)  [unwired: 3 in, 2 out]
                n254 = call "HandleError.vi"("error in (no error)"=w316) -> ()
              }
            }
            n255 = property on="max. F2 Value" class="DigNum (strict)"("Value"=w312) -> ()  [unwired: 2 in, 2 out]
            n256 = property on="min. F2 Value" class="DigNum (strict)"("Value"=w313) -> ()  [unwired: 2 in, 2 out]
          }
          event #8 {
            n257 = event-data() -> ()  [unwired: 1 in, 5 out]
            n258 = stacked-sequence {
              tunnel: [_ TRUE] -> w334
              frame #0 {
              }
              frame #1 {
              }
            }
          }
          event #9 {
            n259 = event-data() -> ()  [unwired: 1 in, 3 out]
            n260 = event-data("Discard?"=FALSE) -> ()  [unwired: 1 in, 1 out]
          }
        }
      }
    }
    frame #2 {
      n261 = property on="notes" class="String"() -> ("Value"=w351:string)  [unwired: 2 in, 2 out]
      n262 = property class="Str"(reference=w350, "Value"=w351) -> ()  [unwired: 1 in, 2 out]
      n263 = property on="threshold (min)" class="DigNum (strict)"() -> ("Value"=w345:u16)  [unwired: 2 in, 2 out]
      n264 = property on="Color Palette lifetime" class="Enum (strict)"() -> ("Value"=w344:T1)  [unwired: 2 in, 2 out]
      n265 = property on="Color Palette F2-image" class="Enum (strict)"() -> ("Value"=w343:T1)  [unwired: 2 in, 2 out]
      n266 = property on="min. F2 Value" class="DigNum (strict)"() -> ("Value"=w342:sgl)  [unwired: 2 in, 2 out]
      n267 = property on="max. F2 Value" class="DigNum (strict)"() -> ("Value"=w341:sgl)  [unwired: 2 in, 2 out]
      n268 = property on="min. tau Value" class="DigNum (strict)"() -> ("Value"=w340:dbl)  [unwired: 2 in, 2 out]
      n269 = property on="max. tau Value" class="DigNum (strict)"() -> ("Value"=w339:dbl)  [unwired: 2 in, 2 out]
      n270 = call "LifetimeImageglobal.vi"("Enum"=T3."dump") -> ("error out"=w354:errorcluster)  [unwired: 5 in, 2 out]
      n271 = call "F2Imageglobal.vi"("error in"=w354, "Enum"=T2."dump") -> ("error out"=w338:errorcluster)  [unwired: 7 in, 2 out]
      n272 = call "HandleError.vi"("error in (no error)"=w338) -> ()
      n273 = call "StandardSettings.vi"("Enum"=enum16{"Load", "get", "Save", "set"}."get") -> ("StandardSettings"=w348:T8)  [unwired: 4 in]
      n274 = Bundle By Name(cluster=w348, "threshold.min"=w345, "F2-lifetime.Palette Number lifetime"=w344, "F2-lifetime.Palette Number F2"=w343, "F2-lifetime.min F2-Value"=w342, "F2-lifetime.max F2-Value"=w341, "F2-lifetime.min tau-Value"=w340, "F2-lifetime.max tau-Value"=w339) -> (w346:T8)
      n275 = call "StandardSettings.vi"("StandardSettings"=w346, "Enum"=enum16{"Load", "get", "Save", "set"}."set") -> ()  [unwired: 3 in, 1 out]
      n276 = property class="VI"("Front Panel Window:Open"=FALSE) -> ()  [unwired: 2 in, 2 out]
    }
  }
  n277 = property on="Color Palette F2-image" class="Enum (strict)" props=["Value"]() -> ()  [unwired: 2 in, 3 out]
  n278 = property on="F2-channel" class="Digital (strict)" props=["Value"]() -> ()  [unwired: 2 in, 3 out]
